vi "Line Up.vi"(8 "error IO":errorcluster, 10 "Component":T1, 11 "Gantry In":refnum<k24>) -> (0 "error out":errorcluster, 2 "Error?":bool, 3 "Gantry Out":refnum<k24>)   [LabVIEW 2021, in "Component Tray.lvclass"]
uses:
  Component Tray.lvclass
  C:/Program Files (x86)/Aerotech/A3200/LabVIEW/2010/Bin/Aerotech.A3200.dll
  Program Files (x86)/Aerotech/A3200/LabVIEW/2010/Bin/Aerotech.A3200.dll
  Find Component.ctl
  Controller/Camera/Machine Vision.ctl
  Controller/Motion/A3200/A3200.lvclass
  Controller/Camera/Camera.lvclass
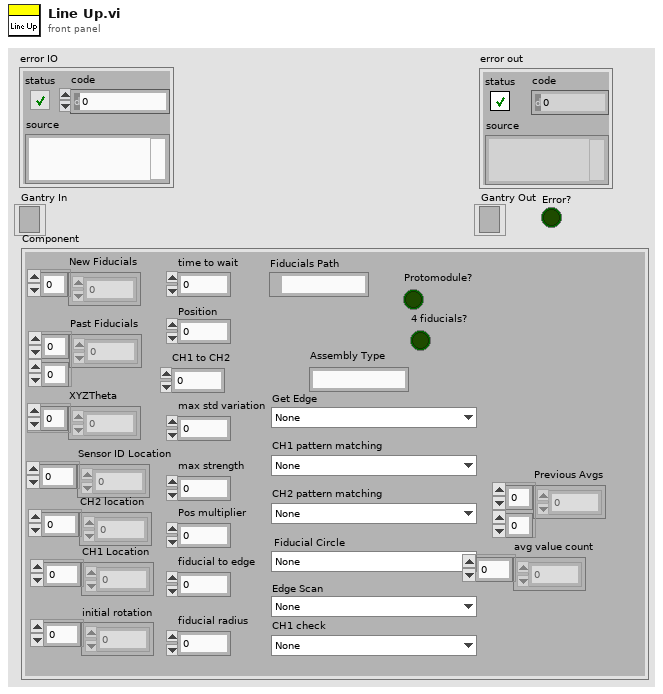
[diagram p1: front panel]
types:
  T1 = typedef "Component Tray.lvclass/Find Component.ctl" = cluster{"New Fiducials":dbl[], "Past Fiducials":dbl[][], "XYZTheta":dbl[], "Fiducials Path":path, "Position":i32, "CH1 Location":dbl[], "Sensor ID Location":dbl[], "initial rotation":dbl[], "CH2 location":dbl[], "max std variation":dbl, "max strength":dbl, "CH2 pattern matching":T2, "Fiducial Circle":T2, "Get Edge":T2, "Pos multiplier":dbl, "time to wait":u32, "fiducial to edge":dbl, "Protomodule?":bool, "Assembly Type":string, "CH1 to CH2":dbl, "Tray Number":string, "fiducial radius":dbl, "4 fiducials?":bool, "CH1 check":T2, "Edge Scan":T2, "CH1 pattern matching":T2, "Sensor Thickness":dbl, "Previous Avgs":dbl[][], "avg value count":dbl[]}
  T2 = typedef "Camera.lvclass/Machine Vision.ctl" = enum16{"None", "Assembly Tray Circle", "Assembly Tray Fiducial", "Partial Hexaboard", "sensor edge init", "HB edge init", "sensor edge pos1", "sensor edge pos2", "HB edge pos1", "HB edge pos2", "Sensor CH1-2", "HB CH1", "HB CH2", "V3 Sensor Circle", "Hexaboard Circle", "sensor CH1 check", "HB CH1 check ", "sensor ID"}
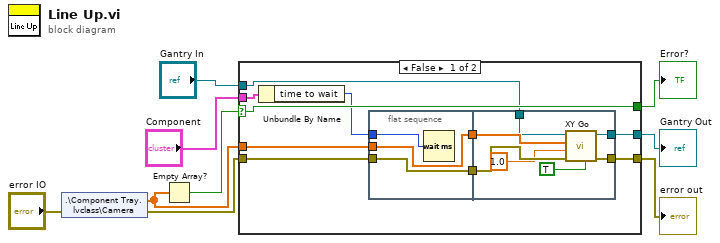
[diagram p0: block diagram]
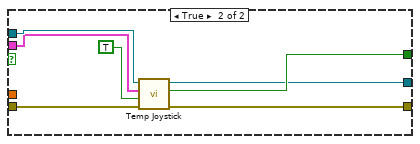
[diagram p2: hidden frame]
diagram:
  n1 = shared-variable ".\\Component Tray.lvclass\\Camera"(error in="error IO") -> (w3:dbl[], error out=w5:errorcluster)
  n2 = Empty Array?(array=w3) -> (empty?=w8:bool)
  n3 = case shown="False" w8 {
    selector: w8 -> [w13 _]
    tunnel: "Gantry In" -> [w12 w36]
    tunnel: "Component" -> [w11 w35]
    tunnel: w5 -> [w14 w33]
    tunnel: [w13 w32] -> w4
    tunnel: w3 -> [w17 _]
    tunnel: [w16 w30] -> w2
    tunnel: [w15 w31] -> w1
    frame False {
      n4 = Unbundle By Name(w11) -> ("time to wait"=w10:u32)
      n5 = flat-sequence {
        tunnel: [w22] -> w19
        tunnel: [w21] -> w18
        tunnel: w14 -> [w22]
        tunnel: w17 -> [w21]
        tunnel: w10 -> [w20]
        tunnel: w19 -> [w28]
        tunnel: w18 -> [w27]
        tunnel: [w26] -> w16
        tunnel: [w25] -> w15
        tunnel: w12 -> [w24]
        frame #0 {
          n6 = Wait (ms)(milliseconds to wait=w20) -> ()  [unwired: 1 out]
        }
        frame #1 {
          n7 = call "XY Go.vi"("Increment?"=TRUE, "error in (no error)"=w28, "Speed"=1.0, "XY In"=w27, "Gantry In"=w24) -> ("error out"=w26:errorcluster, "Gantry Out"=w25:refnum<k24>)  [unwired: 4 in, 1 out]
        }
      }
    }
    frame True {
      n8 = call "Temp Joystick.vi"("error in (no error)"=w33, "Fiducial?"=TRUE, "Component"=w35, "Gantry In"=w36) -> ("error out"=w30:errorcluster, "Error?"=w32:bool, "Gantry Out"=w31:refnum<k24>)  [unwired: 5 in]
    }
  }
  "error out" <- w2
  "Gantry Out" <- w1
  "Error?" <- w4
